vi "Update Check-out Details.vi"(0 "Hotel Management Tool Model in":refnum<class "Hotel Management Tool Model.lvclass">, 5 "Rooms Manager GUID":string, 7 "Bill Summary":string, 11 "error in (no error)":errorcluster) -> (4 "Hotel Management Tool Model out":refnum<class "Hotel Management Tool Model.lvclass">, 15 "error out":errorcluster)   [LabVIEW 2023, in "Hotel Management Tool Model.lvlib" / "Hotel Management Tool Model.lvclass"]
uses:
  Hotel Management Tool Model.lvclass
  Hotel Management Tool Model.lvclass/Hotel Management Tool Model.ctl
  Rooms Manager Model/Rooms Manager Model Messages/Update Check-out Details Msg/Update Check-out Details Msg.lvclass
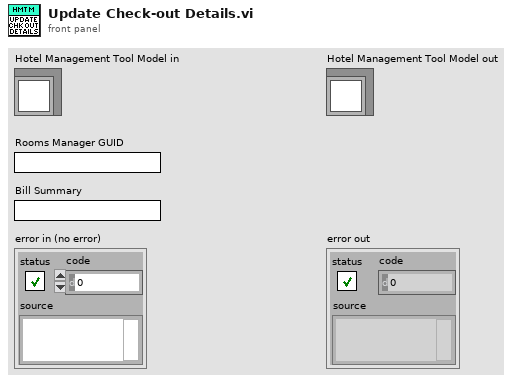
[diagram p1: front panel]
types:
  T1 = map{string, refnum<class "Message Enqueuer.lvclass">}
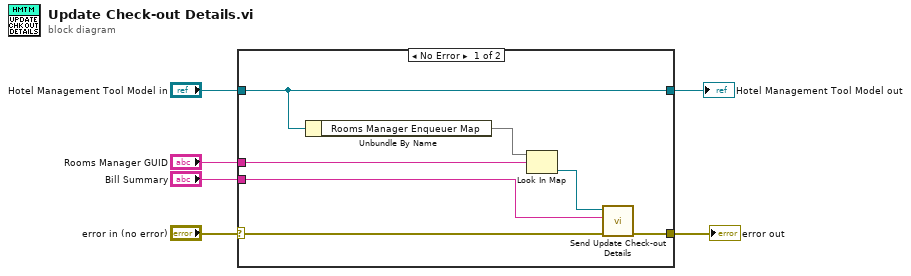
[diagram p0: block diagram]
diagram:
  n1 = case shown="No Error" "error in (no error)" {
    selector: "error in (no error)" -> [w13 w15]
    tunnel: [w12 w15] -> w4
    tunnel: "Hotel Management Tool Model in" -> [w7 w14]
    tunnel: "Rooms Manager GUID" -> [w10 _]
    tunnel: "Bill Summary" -> [w9 _]
    tunnel: [w7 w14] -> w6
    frame No Error {
      n2 = Unbundle By Name(w7) -> ("Rooms Manager Enqueuer Map"=w11:T1)
      n3 = Look In Map(map=w11, key=w10) -> (value=w8:refnum<class "Message Enqueuer.lvclass">)  [unwired: 1 in, 1 out]
      n4 = call "Send Update Check-out Details.vi"("error in (no error)"=w13, "Bill Summary"=w9, "Message Enqueuer"=w8) -> ("error out"=w12:errorcluster)  [unwired: 7 in, 1 out]
    }
    frame Error {
    }
  }
  "error out" <- w4
  "Hotel Management Tool Model out" <- w6
